vi "Create GBs in sequence.vi"() -> ()   [LabVIEW 2010]
uses:
  <vilib>/Utility/file.llb/Write To Spreadsheet File (string).vi
panel:
  in  "Grain Growth and Geometry":T1={"Grain 1 Length (prop)"=1.0, "Grain 2 Length (prop)"=1.0, "Max Grain Height (A)"=80.0, "Max Grain Width (A)"=80.0, "Grain 1 Start"=-0.001, "Overlap Region (A)"=0.001}
  out "Total # of calcs":i32
  in  "Start again index":i32
  out "Array":T2(array[cluster])
  in  "# of Pts":dbl=5.0
  out "# of Reduced":i32
  in  "Relaxation Type":string(combo)="conp opti"
  out "Current Index":i32
  in  "Reduce to Repeating":T3={"Slab X"=4.6, "Slab Y"=4.0, "Tolerance (A)"=0.5, "Presorted?"=FALSE}
  in  "Path":path
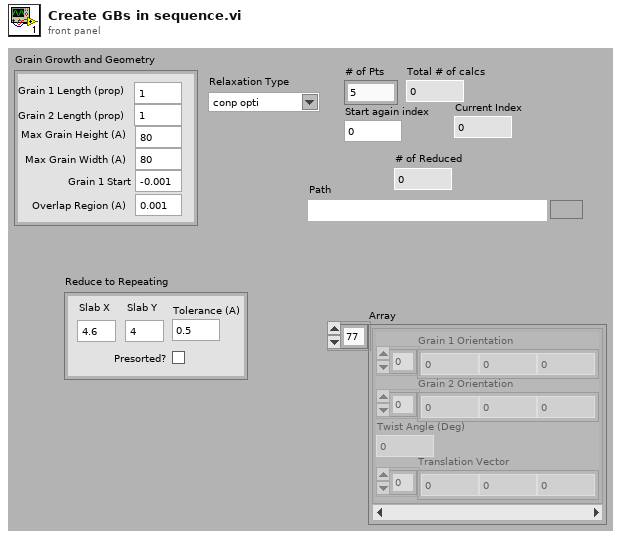
[diagram p1: front panel]
types:
  T1 = cluster{"Grain 1 Length (prop)":dbl, "Grain 2 Length (prop)":dbl, "Max Grain Height (A)":dbl, "Max Grain Width (A)":dbl, "Grain 1 Start":dbl, "Overlap Region (A)":dbl}
  T2 = cluster{"Grain 1 Orientation":dbl[], "Grain 2 Orientation":dbl[], "Twist Angle (Deg)":dbl, "Translation Vector":dbl[]}[]
  T3 = cluster{"Slab X":dbl, "Slab Y":dbl, "Tolerance (A)":dbl, "Presorted?":bool}
  T4 = cluster{"Grain 1 Orientation":dbl[], "Grain 2 Orientation":dbl[], "Twist Angle (Deg)":dbl, "Translation Vector":dbl[]}
  T5 = cluster{"Structure Name":string, "Lattice vector a":dbl[], "Lattice vector b":dbl[], "Lattice vector c":dbl[], "Atoms Array":cluster{"Atom Name":string, "Positions (Direct)":dbl[][], "Positions (Cartesian)":dbl[][]}[], "# of atoms":i32}
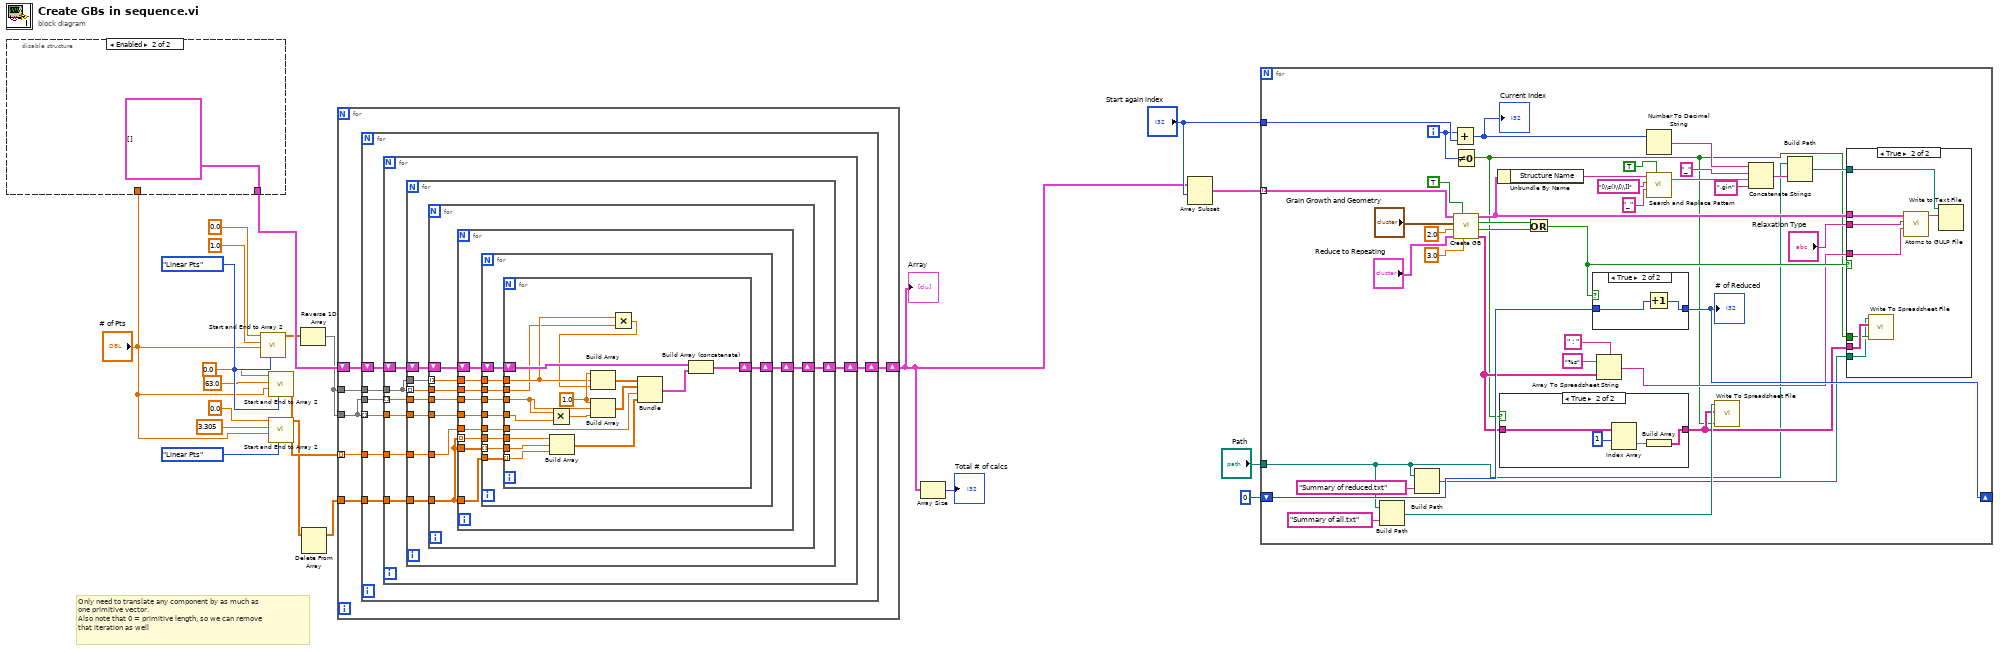
[diagram p0: block diagram]
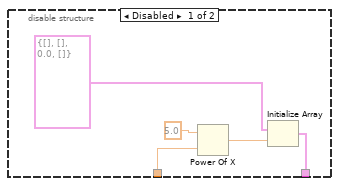
[diagram p2: hidden frame]
diagram:
  w14 = enum16{"Linear Step", "Linear Pts", "Log Pts"}."Linear Pts" ("Sweep Style")
  # "Only need to translate any component by as much as \none primitive vector.\nAlso note that 0 = primitive length, so we can remove\nthat iteration as well"
  n1 = disable-structure shown="Enabled" {
    disable-tunnel: "# of Pts" -> [w26 _]
    disable-tunnel: [w22 T2 []] -> w5
    frame Disabled {
      n2 = Power Of X(1:w26, 2:5.0 ("y")) -> (0:w24:dbl)
      n3 = Initialize Array(T4 {"Grain 1 Orientation"=[], "Grain 2 Orientation"=[], "Twist Angle (Deg)"=0.0, "Translation Vector"=[]} ("Grain Boundary Definition"), w24) -> (w22:T2)
    }
    frame Enabled {
    }
  }
  n4 = call "Start and End to Array 2.vi"("Sweep Style"=w14, "Step or # Pts"="# of Pts", "End"=1.0, "Start"=0.0) -> ("Array"=w2:dbl[])  [unwired: 7 in]
  n5 = call "Start and End to Array 2.vi"("Sweep Style"=w14, "Step or # Pts"="# of Pts", "End"=63.0, "Start"=0.0) -> ("Array"=w11:dbl[])  [unwired: 7 in]
  n6 = call "Start and End to Array 2.vi"("Sweep Style"=enum16{"Linear Step", "Linear Pts", "Log Pts"}."Linear Pts", "Step or # Pts"="# of Pts", "End"=3.305, "Start"=0.0) -> ("Array"=w4:dbl[])  [unwired: 7 in]
  n7 = Reverse 1D Array(array=w2) -> (reversed array=w1:dbl[])
  n8 = Delete From Array(array=w4) -> (array with subset deleted=w3:dbl[])  [unwired: 2 in, 1 out]
  n9 = for {
    tunnel: w3 -> [w33]
    tunnel: w1 -> [w32]
    tunnel: w1 -> [w31]
    tunnel: w11 -> [w30] mode=indexing
    shift-right: [w29] -> w8
    shift-left: w5 -> [w28]
    n10 = for {
      tunnel: w33 -> [w40]
      tunnel: w32 -> [w39]
      tunnel: w31 -> [w38]
      tunnel: w31 -> [w37] mode=indexing
      tunnel: w30 -> [w36]
      shift-right: [w35] -> w29
      shift-left: w28 -> [w34]
      n11 = for {
        tunnel: w40 -> [w47]
        tunnel: w39 -> [w46]
        tunnel: w38 -> [w45] mode=indexing
        tunnel: w37 -> [w44]
        tunnel: w36 -> [w43]
        shift-right: [w42] -> w35
        shift-left: w34 -> [w41]
        n12 = for {
          tunnel: w47 -> [w55]
          tunnel: w46 -> [w54]
          tunnel: w46 -> [w53] mode=indexing
          tunnel: w45 -> [w52]
          tunnel: w44 -> [w51]
          tunnel: w43 -> [w50]
          shift-right: [w49] -> w42
          shift-left: w41 -> [w48]
          n13 = for {
            tunnel: w55 -> [w63]
            tunnel: w54 -> [w62] mode=indexing
            tunnel: w53 -> [w61]
            tunnel: w52 -> [w60]
            tunnel: w51 -> [w59]
            tunnel: w50 -> [w58]
            shift-right: [w57] -> w49
            shift-left: w48 -> [w56]
            n14 = for {
              tunnel: w63 -> [w73]
              tunnel: w63 -> [w72]
              tunnel: w63 -> [w71] mode=indexing
              tunnel: w62 -> [w70]
              tunnel: w61 -> [w69]
              tunnel: w60 -> [w68]
              tunnel: w59 -> [w67]
              tunnel: w58 -> [w66]
              shift-right: [w65] -> w57
              shift-left: w56 -> [w64]
              n15 = for {
                tunnel: w73 -> [w83]
                tunnel: w72 -> [w82] mode=indexing
                tunnel: w71 -> [w81]
                tunnel: w70 -> [w80]
                tunnel: w69 -> [w79]
                tunnel: w68 -> [w78]
                tunnel: w67 -> [w77]
                tunnel: w66 -> [w76]
                shift-right: [w75] -> w65
                shift-left: w64 -> [w74]
                n16 = for {
                  tunnel: w83 -> [w95] mode=indexing
                  tunnel: w82 -> [w96]
                  tunnel: w81 -> [w97]
                  tunnel: w80 -> [w89]
                  tunnel: w79 -> [w88]
                  tunnel: w78 -> [w86]
                  tunnel: w77 -> [w85]
                  tunnel: w76 -> [w93]
                  shift-right: [w91] -> w75
                  shift-left: w74 -> [w90]
                  w99 = 1.0 ("element")
                  n17 = Multiply(x=w86, y=w85) -> (x*y=w84:dbl)
                  n18 = Build Array(w97, w96, w95) -> (w98:dbl[])
                  n19 = Build Array(w99, w86, w84) -> (w94:dbl[])
                  n20 = Multiply(x=w89, y=w88) -> (x*y=w87:dbl)
                  n21 = Build Array(w99, w89, w87) -> (w100:dbl[])
                  n22 = Bundle(w100, w94, w93, w98) -> (w92:cluster{dbl[], dbl[], dbl, dbl[]})  [unwired: 1 in]
                  n23 = Build Array (concatenate)(w90, w92) -> (w91:T2)
                }
              }
            }
          }
        }
      }
    }
  }
  "Array" <- w8
  n24 = Array Size(array=w8) -> (size(s)=→"Total # of calcs":i32)
  n25 = Array Subset(array=w8, index="Start again index") -> (w10:T2)  [unwired: 1 in]
  n26 = for {
    tunnel: "Path" -> [w104]
    shift-right: [w120] -> _
    shift-left: 0 -> [w121]
    tunnel: w10 -> [w117] mode=indexing
    tunnel: "Start again index" -> [w116]
    i -> [w109]
    n27 = Build Path(base path=w104, name or relative path="Summary of all.txt") -> (appended path=w108:path)
    n28 = Build Path(base path=w104, name or relative path="Summary of reduced.txt") -> (appended path=w102:path)
    n29 = Add(x=w109, y=w116) -> (x+y=w115:i32)
    "Current Index" <- w115
    n30 = Not Equal To 0?(x=w109) -> (x != 0?=w105:bool)
    n31 = call "Create GB.vi"("Edge Duplication Range"=3.0, "Skip cleanup if no subset"=TRUE ("Skip crop if no subset"), "Reduce to Repeating"="Reduce to Repeating", "Min Seperation Distance (A)"=2.0, "Grain Growth and Geometry"="Grain Growth and Geometry", "Grain Boundary Definition"=w117) -> ("GB Data"=w107:string[][], "Reduced Orthorhombic?"=w122:bool, "Reduced Rhombahedral?"=w123:bool, "Grain Boundary"=w137:T5)  [unwired: 1 in, 1 out]
    n32 = Unbundle By Name(w137) -> ("Structure Name"=w126:string)
    n33 = case shown="True" w105 {
      tunnel: [w138 w139] -> w106
      tunnel: w107 -> [w138 w142]
      frame False {
      }
      frame True {
        n34 = Index Array(array=w142, index (row)=1) -> (element=w140:string[])  [unwired: 1 in]
        n35 = Build Array(w140) -> (w139:string[][])
      }
    }
    n36 = Or(x=w123, y=w122) -> (x .or. y?=w119:bool)
    n37 = case shown="True" w119 {
      tunnel: w121 -> [w151 w153]
      tunnel: [w151 w152] -> w120
      frame False {
      }
      frame True {
        n38 = Increment(x=w153) -> (x+1=w152:i32)
      }
    }
    "# of Reduced" <- w120
    n39 = Array To Spreadsheet String(delimiter (Tab)=" : ", array=w107, 3:"%s" ("format string")) -> (spreadsheet string=w111:string)
    n40 = Number To Decimal String(number=w115) -> (decimal integer string=w136:string)  [unwired: 1 in]
    n41 = call <vilib>:"Search and Replace Pattern.vi"("string"=w126, "regular expression (\"\")"="[\\s()\\[\\]]" ("regular expression (\"\")"), "replace string (\"\")"="_" ("replace string (\"\")"), "replace all? (F)"=TRUE) -> ("result string"=w125:string)  [unwired: 1 in, 1 out]
    n42 = call-poly <vilib>:"Write To Spreadsheet File.vi"("append to file? (new file:F)"=w105, "2D data"=w106, "file path (dialog if empty)"=w108) -> ()  [unwired: 5 in, 1 out]
    n43 = Concatenate Strings(w136, "_" ("string"), w125, ".gin" ("string")) -> (w135:string)
    n44 = Build Path(base path=w104, name or relative path=w135) -> (appended path=w134:path)
    n45 = case shown="True" w119 {
      tunnel: w137 -> [_ w150]
      tunnel: w134 -> [_ w149]
      tunnel: "Relaxation Type" -> [_ w148]
      tunnel: w111 -> [_ w146]
      tunnel: w106 -> [_ w145]
      tunnel: w105 -> [_ w144]
      tunnel: w102 -> [_ w143]
      frame False {
      }
      frame True {
        n46 = call-poly <vilib>:"Write To Spreadsheet File.vi"("append to file? (new file:F)"=w144, "2D data"=w145, "file path (dialog if empty)"=w143) -> ()  [unwired: 5 in, 1 out]
        n47 = call "Atoms to GULP File.vi"("Title and Comments"=w146, "Relaxation Type"=w148, "Structure"=w150) -> ("GULP File"=w147:string)  [unwired: 8 in]
        n48 = Write to Text File(file (use dialog)=w149, text=w147) -> ()  [unwired: 2 in, 3 out]
      }
    }
  }
